vi "Clear Data.vi"(8 "error in (no error)":errorcluster, 11 "TriggerAction in":refnum<class "TriggerAction Q.lvclass">) -> (0 "error out":errorcluster, 3 "TriggerAction out":refnum<class "TriggerAction Q.lvclass">)   [LabVIEW 2016, in "TriggerAction Q.lvclass"]
uses:
  <userlib>/Common Components/TriggerAction Q/TriggerAction Q/TriggerAction Q.lvclass
  <userlib>/Common Components/TriggerAction Q/TriggerAction Q/TriggerAction Q.lvclass/TriggerAction Q.ctl
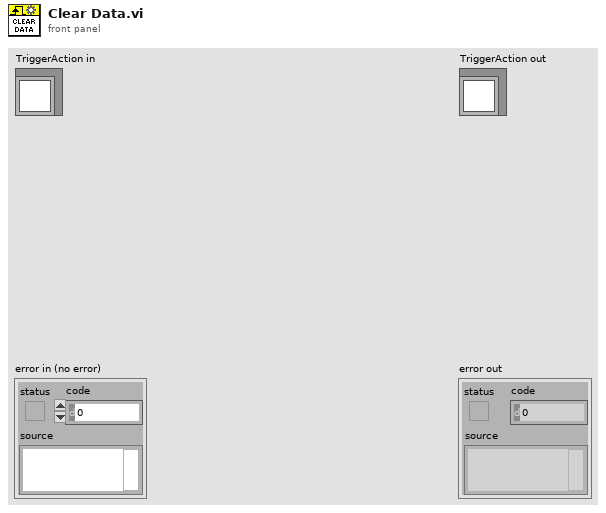
[diagram p1: front panel]
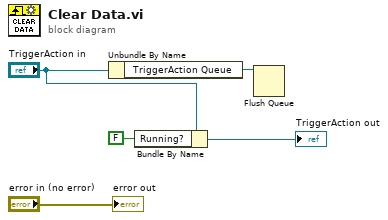
[diagram p0: block diagram]
diagram:
  n1 = Unbundle By Name("TriggerAction in") -> ("TriggerAction Queue"=w3:refnum<queue>)
  n2 = Bundle By Name(cluster="TriggerAction in", "Running?"=FALSE) -> (→"TriggerAction out":refnum<class "TriggerAction Q.lvclass">)
  n3 = Flush Queue(queue=w3) -> ()  [unwired: 1 in, 3 out]
  "error out" <- "error in (no error)"
